vi "Read Sensor Init Complete.vi"(0 "FPGA VI Reference in":T1, 3 "error in (no error)":errorcluster) -> (7 "FPGA VI Reference out":T1, 8 "Initialization Complete":bool, 10 "error out":errorcluster)   [LabVIEW 2009]
uses:
  TypeDefs/Sensor Typedefs/FPGA Main ref.ctl
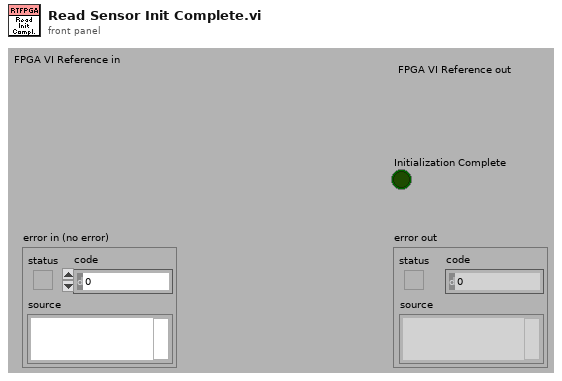
[diagram p1: front panel]
types:
  T1 = typedef "FPGA Main ref.ctl" = refnum<k20>
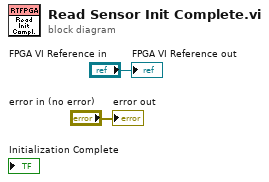
[diagram p0: block diagram]
diagram:
  "FPGA VI Reference out" <- "FPGA VI Reference in"
  "error out" <- "error in (no error)"
